vi "Init.vi"(7 "Sender":refnum<class "Sender.lvclass">) -> (3 "Go To Destroy Msg out":refnum<class "Go To Destroy Msg.lvclass">)   [LabVIEW 2020, in "jettl.lvlib" / "Go To Destroy Msg.lvlib" / "Go To Destroy Msg.lvclass"]
uses:
  Go To Destroy Msg.lvclass
  Sender/Sender/Sender.lvclass
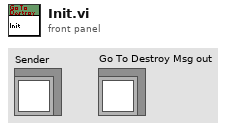
[diagram p1: front panel]
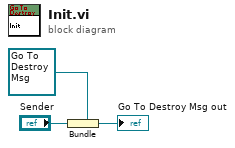
[diagram p0: block diagram]
diagram:
  n1 = Bundle "Bundle"(cluster=refnum<class "Go To Destroy Msg.lvclass"> refnum ("Destroy Msg in"), "Sender") -> (→"Go To Destroy Msg out":refnum<class "Go To Destroy Msg.lvclass">)
